vi "W7X1DPut.vi"(0 "SigLabel":string="MTau", 2 "Unit":string="s", 5 "SigJSONbuffer":string, 9 "values":T1(array[cluster]), 11 "local storage only":bool, 14 "dimensions":i64[](array[numeric])=[1428413878000000000, -1]) -> (3 "body":string, 4 "body Parlog":string, 6 "headers parms":string, 10 "file path written":string, 12 "headers":string, 15 "Parlog error out":errorcluster)   [LabVIEW 2014]
uses:
  <vilib>/httpClient/POSTBuffer.vi
  <vilib>/httpClient/LabVIEWHTTPClient.lvlib
panel:
  out "JSON string":string
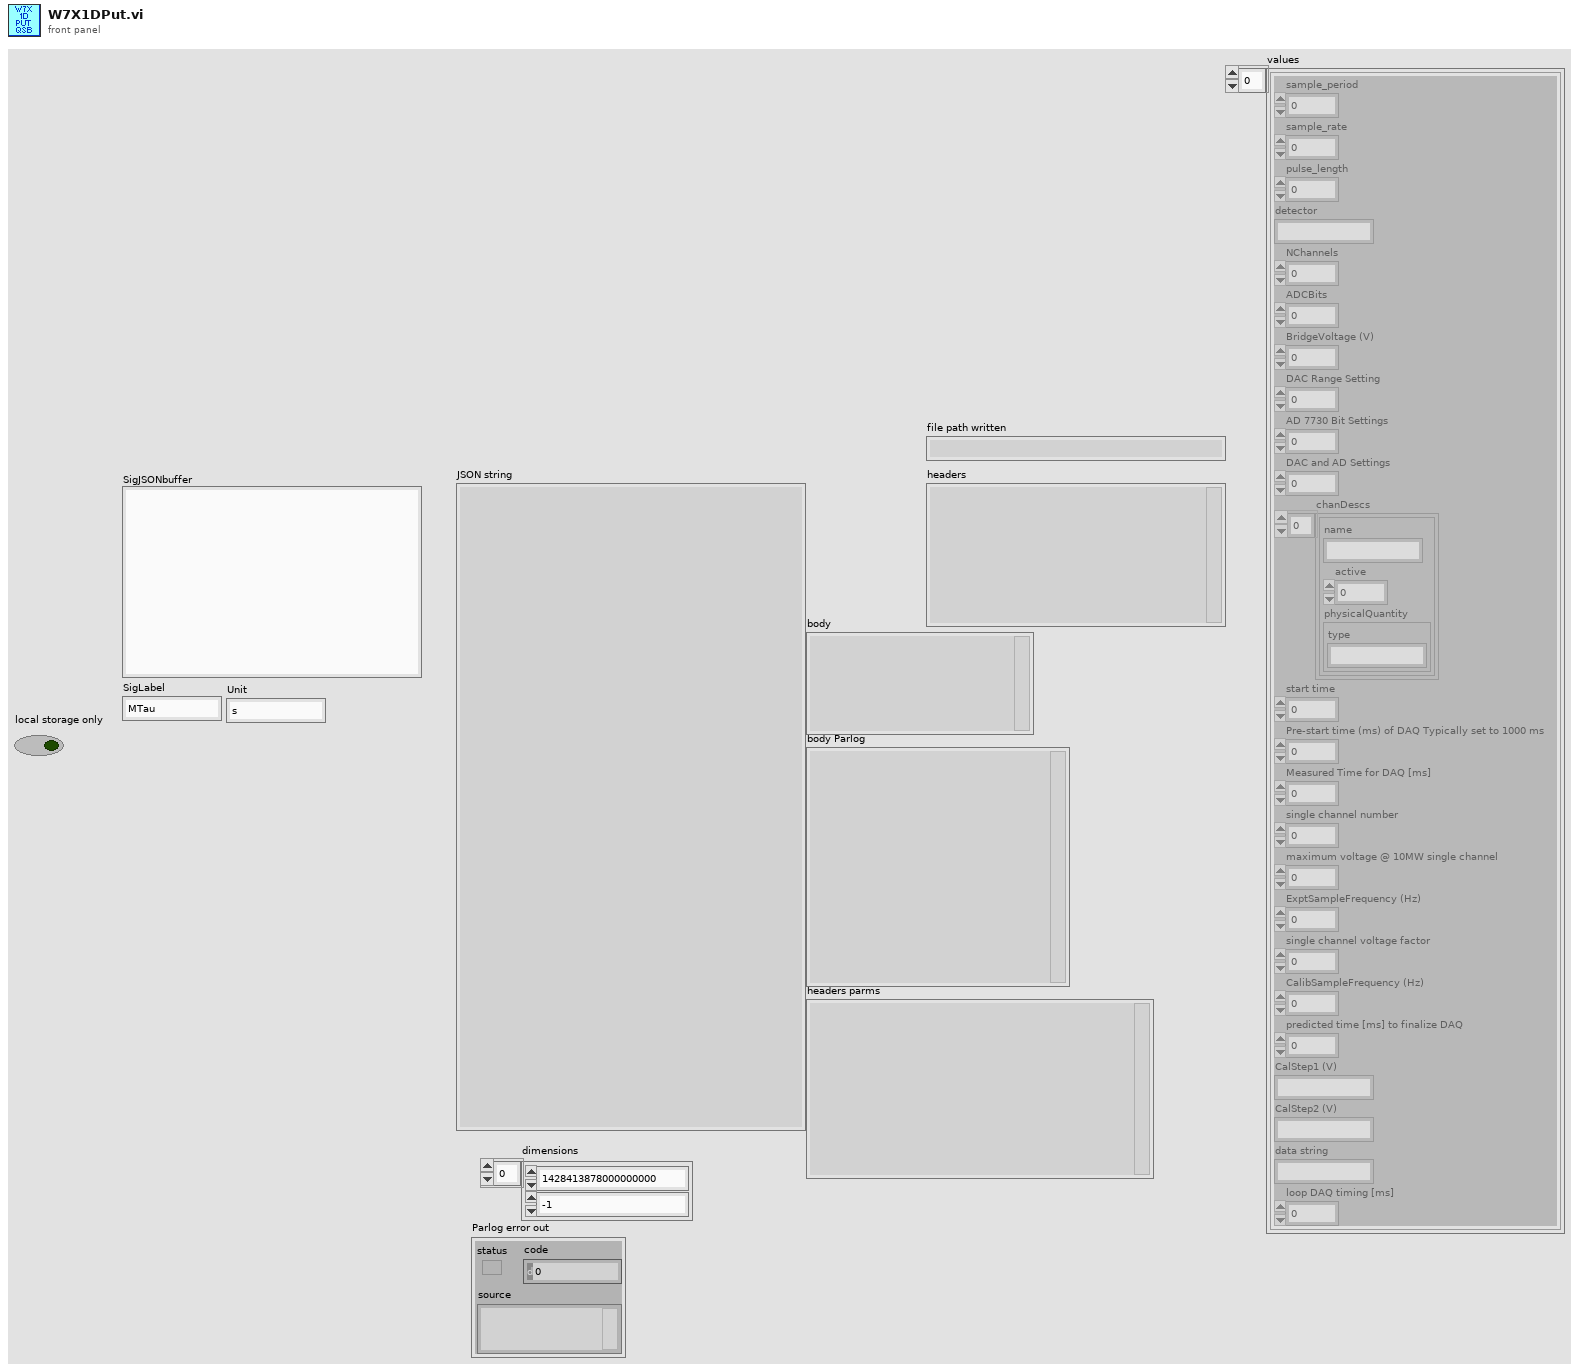
[diagram p1: front panel]
types:
  T1 = cluster{"sample_period":dbl, "sample_rate":dbl, "pulse_length":dbl, "detector":string, "NChannels":i16, "ADCBits":i16, "BridgeVoltage (V)":sgl, "DAC Range Setting":u8, "AD 7730 Bit Settings":i32, "DAC and AD Settings":i32, "chanDescs":cluster{"name":string, "active":i32, "physicalQuantity":cluster{"type":string}}[], "start time":i64, "Pre-start time (ms) of DAQ Typically set to 1000 ms":i32, "Measured Time for DAQ [ms] ":u32, "single channel number":i64, "maximum voltage @ 10MW single channel":dbl, "ExptSampleFrequency (Hz)":sgl, "single channel voltage factor":dbl, "CalibSampleFrequency (Hz)":sgl, "predicted time [ms] to finalize DAQ":dbl, "CalStep1 (V)":string, "CalStep2 (V)":string, "data string":string, "loop DAQ timing [ms]":dbl}[]
  T2 = cluster{"sample_period":dbl, "sample_rate":dbl, "pulse_length":dbl, "detector":string, "NChannels":i16, "ADCBits":i16, "BridgeVoltage (V)":sgl, "DAC Range Setting":u8, "AD 7730 Bit Settings":i32, "DAC and AD Settings":i32, "chanDescs":cluster{"name":string, "active":i32, "physicalQuantity":cluster{"type":string}}[], "start time":i64, "Pre-start time (ms) of DAQ Typically set to 1000 ms":i32, "Measured Time for DAQ [ms] ":u32, "single channel number":i64, "maximum voltage @ 10MW single channel":dbl, "ExptSampleFrequency (Hz)":sgl, "single channel voltage factor":dbl, "CalibSampleFrequency (Hz)":sgl, "predicted time [ms] to finalize DAQ":dbl, "CalStep1 (V)":string, "CalStep2 (V)":string, "data string":string, "loop DAQ timing [ms]":dbl}
  T3 = cluster{"name":string, "active":i32, "physicalQuantity":cluster{"type":string}}[]
  T4 = cluster{"name":string, "active":i32, "physicalQuantity":cluster{"type":string}}
  T5 = cluster{"label":string, "values":cluster{"sample_period":dbl, "sample_rate":dbl, "pulse_length":dbl, "detector":string, "NChannels":i16, "ADCBits":i16, "BridgeVoltage (V)":sgl, "DAC Range Setting":u8, "AD 7730 Bit Settings":i32, "DAC and AD Settings":i32, "chanDescs":cluster{"name":string, "active":i32, "physicalQuantity":cluster{"type":string}}[], "start time":i64, "Pre-start time (ms) of DAQ Typically set to 1000 ms":i32, "Measured Time for DAQ [ms] ":u32, "single channel number":i64, "maximum voltage @ 10MW single channel":dbl, "ExptSampleFrequency (Hz)":sgl, "single channel voltage factor":dbl, "CalibSampleFrequency (Hz)":sgl, "predicted time [ms] to finalize DAQ":dbl, "CalStep1 (V)":string, "CalStep2 (V)":string, "data string":string, "loop DAQ timing [ms]":dbl}[], "dimensions":i64[]}
  T6 = typedef "LabVIEWHTTPClient.lvlib/ClientHandle.ctl" = refnum<k1>
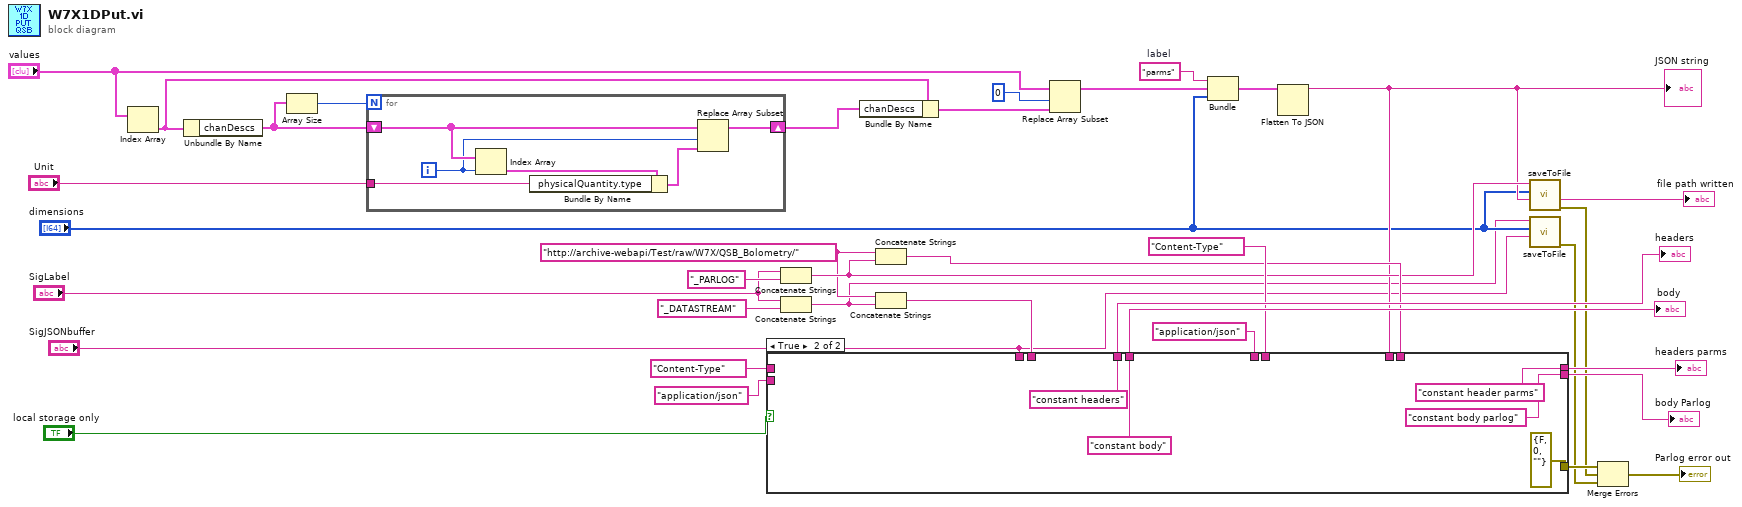
[diagram p0: block diagram]
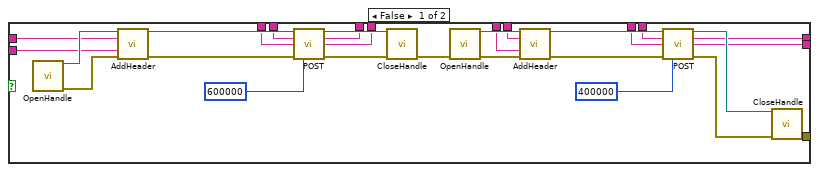
[diagram p2: hidden frame]
diagram:
  w31 = "parms"  # label
  w14 = "http://archive-webapi/Test/raw/W7X/QSB_Bolometry/" ("url")
  n1 = Index Array(array="values") -> (element=w9:T2)  [unwired: 1 in]
  n2 = Unbundle By Name(w9) -> ("chanDescs"=w5:T3)
  n3 = Array Size(array=w5) -> (size(s)=w4:i32)
  n4 = for {
    N: w4 -> [_]
    tunnel: "Unit" -> [w42]
    shift-right: [w38] -> w6
    shift-left: w5 -> [w40]
    i -> [w37]
    n5 = Index Array(array=w40, index=w37) -> (element=w41:T4)
    n6 = Bundle By Name(cluster=w41, "physicalQuantity.type"=w42) -> (w39:T4)
    n7 = Replace Array Subset(array=w40, new element=w39, index=w37) -> (w38:T3)
  }
  n8 = Concatenate Strings("SigLabel", "_PARLOG" ("replace string (\"\")")) -> (w18:string)
  n9 = Concatenate Strings("SigLabel", "_DATASTREAM" ("string")) -> (w13:string)
  n10 = Bundle By Name(cluster=w9, "chanDescs"=w6) -> (w8:T2)
  n11 = Concatenate Strings(w14, w18) -> (w19:string)
  n12 = Concatenate Strings(w14, w13) -> (w15:string)
  n13 = Replace Array Subset(array="values", new element=w8, index=0) -> (w29:T1)
  n14 = Bundle("label"=w31, "values"=w29, "dimensions"="dimensions") -> (w30:T5)  [unwired: 1 in]
  n15 = Flatten To JSON(anything=w30) -> (JSON string=w17:string)  [unwired: 2 in, 1 out]
  "JSON string" <- w17
  n16 = case shown="True" "local storage only" {
    tunnel: [w68 "constant headers" ("headers")] -> w36
    tunnel: "Content-Type" ("header") -> [w63 _]
    tunnel: "application/json" ("value") -> [w62 _]
    tunnel: [w61 "constant body" ("body")] -> w33
    tunnel: [w57 "constant header parms" ("headers")] -> w28
    tunnel: "Content-Type" ("header") -> [w52 _]
    tunnel: "application/json" ("value") -> [w51 _]
    tunnel: [w50 "constant body parlog" ("body")] -> w25
    tunnel: [w48 errorcluster {"status"=FALSE, "code"=0, "source"=""} ("error out")] -> w24
    tunnel: w19 -> [w47 _]
    tunnel: w17 -> [w46 _]
    tunnel: w15 -> [w45 _]
    tunnel: "SigJSONbuffer" -> [w43 _]
    frame False {
      n17 = call <vilib>:"OpenHandle.vi"() -> ("client handle out"=w67:T6, "error out"=w66:errorcluster)  [unwired: 14 in]
      n18 = call <vilib>:"AddHeader.vi"("client handle"=w67, "header"=w63, "value"=w62, "error in (no error)"=w66) -> ("client handle out"=w65:T6, "error out"=w64:errorcluster)  [unwired: 10 in]
      n19 = call-poly <vilib>:"POST.vi"("client handle"=w65, "url"=w45, "buffer"=w43, "error in (no error)"=w64, "timeout (10000)"=600000) -> ("client handle out"=w70:T6, "headers"=w68:string, "body"=w61:string, "error out"=w69:errorcluster)  [unwired: 7 in]
      n20 = call <vilib>:"CloseHandle.vi"("client handle"=w70, "error in (no error)"=w69) -> ("error out"=w44:errorcluster)  [unwired: 13 in]
      n21 = call <vilib>:"OpenHandle.vi"("error in (no error)"=w44) -> ("client handle out"=w56:T6, "error out"=w55:errorcluster)  [unwired: 13 in]
      n22 = call <vilib>:"AddHeader.vi"("client handle"=w56, "header"=w52, "value"=w51, "error in (no error)"=w55) -> ("client handle out"=w54:T6, "error out"=w53:errorcluster)  [unwired: 10 in]
      n23 = call-poly <vilib>:"POST.vi"("client handle"=w54, "url"=w47, "buffer"=w46, "error in (no error)"=w53, "timeout (10000)"=400000) -> ("client handle out"=w59:T6, "headers"=w57:string, "body"=w50:string, "error out"=w58:errorcluster)  [unwired: 7 in]
      n24 = call <vilib>:"CloseHandle.vi"("client handle"=w59, "error in (no error)"=w58) -> ("error out"=w48:errorcluster)  [unwired: 13 in]
    }
    frame True {
    }
  }
  "headers" <- w36
  "body" <- w33
  "headers parms" <- w28
  "body Parlog" <- w25
  n25 = call "saveToFile.vi"("SigJSONbuffer"=w17, "dimensions"="dimensions", "String"=w18) -> ("error out"=w20:errorcluster, "resulting string"=→"file path written":string)  [unwired: 7 in]
  n26 = call "saveToFile.vi"("SigJSONbuffer"="SigJSONbuffer", "dimensions"="dimensions", "String"=w13) -> ("error out"=w12:errorcluster)  [unwired: 7 in, 1 out]
  n27 = Merge Errors(w24, w20, w12) -> (→"Parlog error out":errorcluster)
